vi "Main.vi"() -> ()   [LabVIEW 2019]
uses:
  <vilib>/DAQmx/read.llb/DAQmx Read (Analog DBL 1Chan 1Samp).vi
  <vilib>/DAQmx/create/channels.llb/DAQmx Create Channel (AI-Temperature-Thermocouple).vi
  <vilib>/DAQmx/configure/timing.llb/DAQmx Timing (Sample Clock).vi
  <vilib>/DAQmx/miscellaneous.llb/DAQmx Fill In Error Info.vi
panel:
  in  "maximum value":dbl=100.0 format="%#_13g"
  in  "minimum value":dbl format="%#_13g"
  in  "Stop":bool
  out "Waveform Chart":dbl(graph)
  in  "Thermocouple Channel":tag="PCI-6221/ai0"
  # "Measurement Range (deg C)"
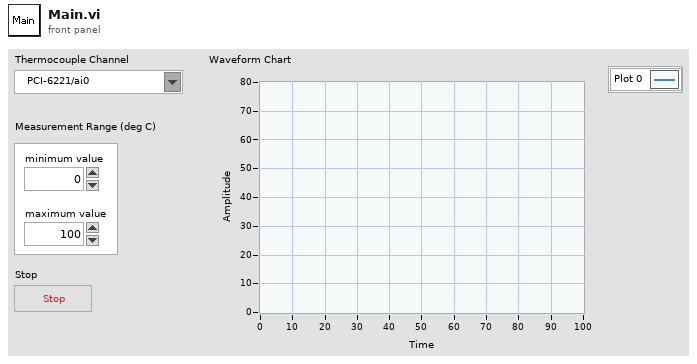
[diagram p1: front panel]
types:
  T1 = enum16{"open", "replace", "create", "open or create", "replace or create", "replace or create with confirmation"}
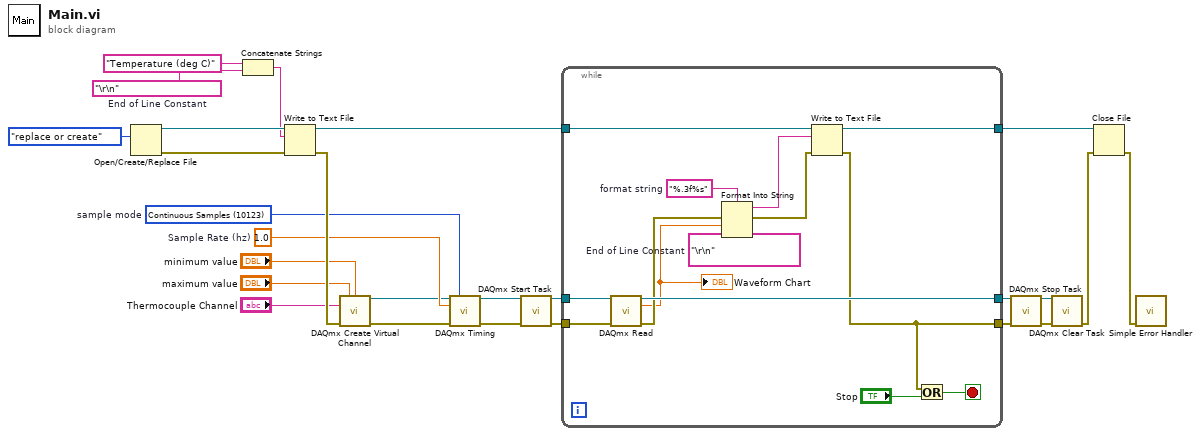
[diagram p0: block diagram]
diagram:
  w10 = "\r\n"  # End of Line Constant
  w24 = 1.0  # Sample Rate (hz)
  w25 = 10123 items=["Finite Samples"=10178, "Continuous Samples"=10123, "Hardware Timed Single Point"=12522]  # sample mode
  n1 = Open/Create/Replace File(operation (0:open)=T1."replace or create") -> (refnum out=w13:refnum<file>, error out=w12:errorcluster)  [unwired: 5 in, 1 out]
  n2 = Concatenate Strings("Temperature (deg C)" ("string"), w10) -> (w9:string)
  n3 = Write to Text File(file (use dialog)=w13, text=w9, error in=w12) -> (refnum out=w8:refnum<file>, error out=w26:errorcluster)  [unwired: 1 in, 1 out]
  n4 = call-poly <vilib>:"DAQmx Create Virtual Channel.vi"("maximum value"="maximum value", "minimum value"="minimum value", "physical channels"="Thermocouple Channel", "error in"=w26) -> ("task out"=w23:refnum<k21>, "error out"=w22:errorcluster)  [unwired: 10 in]
  n5 = call-poly <vilib>:"DAQmx Timing.vi"("task/channels in"=w23, "sample mode"=w25, "rate"=w24, "error in"=w22) -> ("task out"=w21:refnum<k21>, "error out"=w20:errorcluster)  [unwired: 10 in]
  n6 = call <vilib>:"DAQmx Start Task.vi"("task/channels in"=w21, "error in"=w20) -> ("task out"=w16:refnum<k21>, "error out"=w15:errorcluster)  [unwired: 12 in]
  n7 = while {
    tunnel: [w40] -> w7
    tunnel: w16 -> [w37]
    tunnel: w15 -> [w36]
    tunnel: w8 -> [w29]
    tunnel: [w28] -> w6
    tunnel: [w27] -> w2
    stop <- w38 stop-if-true
    w32 = "%.3f%s"  # format string
    w35 = "\r\n"  # End of Line Constant
    n8 = call-poly <vilib>:"DAQmx Read.vi"("task/channels in"=w37, "error in"=w36) -> ("task out"=w40:refnum<k21>, "data"=w33:dbl, "error out"=w34:errorcluster)  [unwired: 11 in]
    "Waveform Chart" <- w33
    n9 = Format Into String(format string=w32, error in=w34, w33, w35) -> (resulting string=w31:string, error out=w30:errorcluster)  [unwired: 1 in]
    n10 = Write to Text File(file (use dialog)=w29, text=w31, error in=w30) -> (refnum out=w27:refnum<file>, error out=w28:errorcluster)  [unwired: 1 in, 1 out]
    n11 = Or(x=w28, y="Stop") -> (x .or. y?=w38:bool)
  }
  n12 = call <vilib>:"DAQmx Stop Task.vi"("task/channels in"=w7, "error in"=w6) -> ("task out"=w5:refnum<k21>, "error out"=w4:errorcluster)  [unwired: 12 in]
  n13 = call <vilib>:"DAQmx Clear Task.vi"("task in"=w5, "error in"=w4) -> ("error out"=w3:errorcluster)  [unwired: 13 in]
  n14 = Close File(refnum=w2, error in=w3) -> (error out=w1:errorcluster)  [unwired: 1 out]
  n15 = call <vilib>:"Simple Error Handler.vi"("error in (no error)"=w1) -> ()  [unwired: 4 in, 5 out]
